vi "whereami.vi"() -> ()   [LabVIEW 2015]
uses:
  G_NAV.vi
  G_VEH.vi
  G_PATH.vi
panel:
  out "Array 2":i32[](array[numeric])
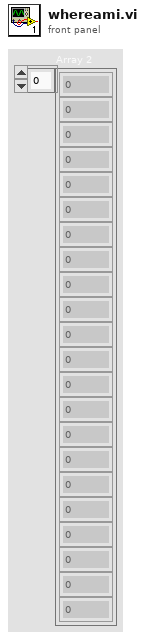
[diagram p1: front panel]
types:
  T1 = cluster{"c_idx":i32, "xc":dbl, "yc":dbl, "hc":dbl, "xc_path":dbl}
  T2 = cluster{"GPSTime":dbl, "attitude[2]":dbl, "lcc[0]":dbl, "lcc[1]":dbl, "heading_GPS":dbl}
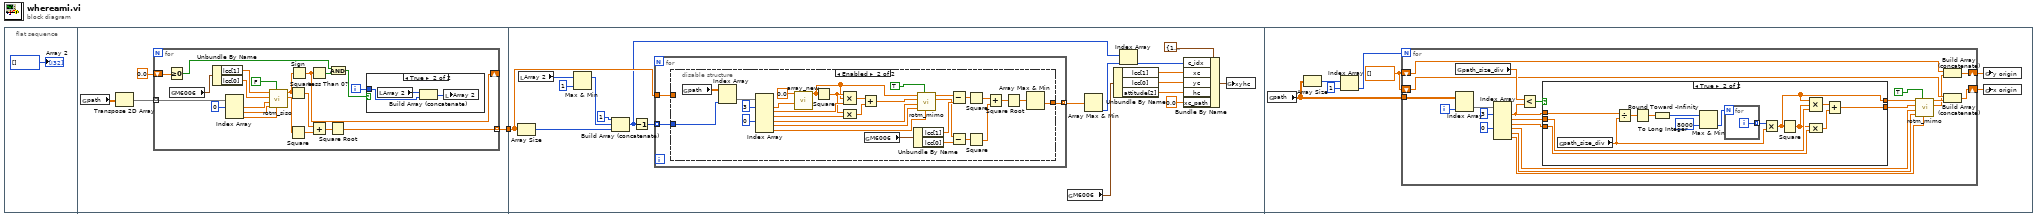
[diagram p0: block diagram]
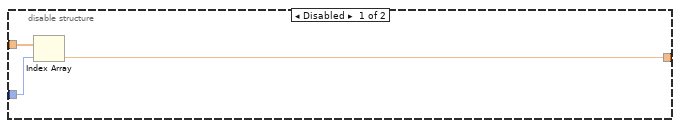
[diagram p3: hidden frame]
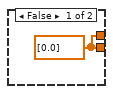
[diagram p4: hidden frame]
diagram:
  n1 = flat-sequence {
    tunnel: [w4] -> w1
    tunnel: w1 -> [w46]
    frame #0 {
      "Array 2" <- i32[] []
    }
    frame #1 {
      n2 = global read "G_PATH.vi" "path"() -> (w3:dbl[][])
      n3 = Transpose 2D Array(2D array=w3) -> (transposed array=w6:dbl[][])
      n4 = for {
        tunnel: w6 -> [w27] mode=indexing
        shift-right: [w13] -> _
        shift-left: 0.0 -> [w18]
        tunnel: [w7] -> w4 mode=indexing
        i -> [w14]
        n5 = Greater Or Equal To 0?(x=w18) -> (x >= 0?=w16:bool)
        n6 = global read "G_NAV.vi" "M6006"() -> (w25:T2)
        n7 = Unbundle By Name(w25) -> ("lcc[1]"=w24:dbl, "lcc[0]"=w23:dbl)
        n8 = Index Array(array=w27, index #1=0 ("index")) -> (element #1=w22:dbl, element #2=w21:dbl, element #3=w20:dbl)  [unwired: 2 in]
        n9 = call "rotm_siso.vi"("angle[rad]"=w20, "reverse"=FALSE, "y0"=w21, "x0"=w22, "y"=w23, "x"=w24) -> ("y'"=w11:dbl, "x'"=w12:dbl)  [unwired: 4 in]
        n10 = Square(x=w12) -> (x^2=w9:dbl)
        n11 = Square(x=w11) -> (x^2=w10:dbl)
        n12 = Sign(1:w12) -> (0:w13:dbl)
        n13 = Less Than 0?(x=w13) -> (x < 0?=w17:bool)
        n14 = Add(x=w9, y=w10) -> (x+y=w8:dbl)
        n15 = Square Root(x=w8) -> (sqrt(x)=w7:dbl)
        n16 = And(x=w16, y=w17) -> (x .and. y?=w15:bool)
        n17 = case shown="True" w15 {
          tunnel: w14 -> [_ w28]
          frame False {
          }
          frame True {
            n18 = local read "Array 2"() -> (w30:i32[])
            n19 = Build Array (concatenate)(w30, w28) -> (w29:i32[])
            n20 = local write "Array 2"(w29) -> ()
          }
        }
      }
    }
    frame #2 {
      n21 = Array Size(array=w46) -> (size(s)=w47:i32)
      n22 = local read "Array 2"() -> (w32:i32[])
      n23 = Max & Min(x=w32, y=1) -> (max(x,y)=w31:i32[])  [unwired: 1 out]
      n24 = Build Array (concatenate)(1 ("y"), w31, w47) -> (w43:i32[])
      n25 = Decrement(x=w43) -> (x-1=w45:i32[])
      n26 = for {
        tunnel: w46 -> [w51]
        tunnel: w45 -> [w50] mode=indexing
        tunnel: [w49] -> w44 mode=indexing
        n27 = disable-structure shown="Enabled" {
          disable-tunnel: w51 -> [w54 _]
          disable-tunnel: w50 -> [w53 w56]
          disable-tunnel: [w52 w59] -> w49
          frame Disabled {
            n28 = Index Array(array=w54, index=w53) -> (element=w52:dbl)
          }
          frame Enabled {
            n29 = global read "G_PATH.vi" "path"() -> (w55:dbl[][])
            n30 = Index Array(array=w55, index (col)=w56) -> (element=w84:dbl[])  [unwired: 1 in]
            n31 = Index Array(array=w84, index #1=3 ("index"), index #4=0 ("index")) -> (element #1=w81:dbl, element #2=w80:dbl, element #3=w78:dbl, element #4=w72:dbl, element #5=w71:dbl, element #6=w60:dbl)  [unwired: 4 in]
            n32 = call "array_new.vi"("end"=w81, "start"=0.0) -> ("Array"=w61:dbl[])  [unwired: 8 in, 1 out]
            n33 = Square(x=w61) -> (x^2=w79:dbl[])
            n34 = Compound Arithmetic op=MULTIPLY(w79, w61, w80) -> (w77:dbl[])
            n35 = Compound Arithmetic op=MULTIPLY(w79, w78) -> (w76:dbl[])
            n36 = Add(x=w77, y=w76) -> (x+y=w74:dbl[])
            n37 = global read "G_NAV.vi" "M6006"() -> (w70:T2)
            n38 = Unbundle By Name(w70) -> ("lcc[1]"=w69:dbl, "lcc[0]"=w68:dbl)
            n39 = call "rotm_mimo.vi"("angle[rad]"=w60, "reverse"=TRUE, "y0"=w71, "x0"=w72, "y"=w74, "x"=w61) -> ("Y"=w62:dbl[], "X"=w63:dbl[])  [unwired: 2 in, 2 out]
            n40 = Subtract(x=w63, y=w69) -> (x-y=w67:dbl[])
            n41 = Subtract(x=w62, y=w68) -> (x-y=w66:dbl[])
            n42 = Square(x=w67) -> (x^2=w65:dbl[])
            n43 = Square(x=w66) -> (x^2=w64:dbl[])
            n44 = Add(x=w65, y=w64) -> (x+y=w58:dbl[])
            n45 = Square Root(x=w58) -> (sqrt(x)=w57:dbl[])
            n46 = Array Max & Min(array=w57) -> (min value=w59:dbl)  [unwired: 3 out]
          }
        }
      }
      n47 = global read "G_NAV.vi" "M6006"() -> (w38:T2)
      n48 = Array Max & Min(array=w44) -> (min index (indices)=w42:i32)  [unwired: 3 out]
      n49 = Unbundle By Name(w38) -> ("lcc[1]"=w37:dbl, "lcc[0]"=w36:dbl, "attitude[2]"=w35:dbl)
      n50 = Index Array(array=w43, index=w42) -> (element=w39:i32)
      n51 = Bundle By Name(cluster=T1 {"c_idx"=1, "xc"=7.6063100382766855, "yc"=-606.4633590892067, "hc"=0.5767419779046403, "xc_path"=-34.68881211625345} ("xyhc"), "c_idx"=w39, "xc"=w37, "yc"=w36, "hc"=w35, "xc_path"=0.0) -> (w41:T1)
      n52 = global write "G_VEH.vi" "xyhc"(w41) -> ()
    }
    frame #3 {
      w89 = dbl[] []
      n53 = global read "G_PATH.vi" "path"() -> (w85:dbl[][])
      n54 = Array Size(array=w85) -> (size(s)=w88:i32[])
      n55 = Index Array(array=w88, index=1) -> (element=w86:i32)
      n56 = for {
        N: w86 -> [_]
        shift-right: [w97] -> w90
        shift-left: w89 -> [w99]
        shift-right: [w94] -> w91
        shift-left: w89 -> [w96]
        tunnel: w85 -> [w92]
        i -> [w93]
        n57 = global read "G_VEH.vi" "path_size_div"() -> (w108:dbl)
        n58 = Index Array(array=w92, index (col)=w93) -> (element=w113:dbl[])  [unwired: 1 in]
        n59 = Index Array(array=w113, index #1=3 ("index"), index #4=0 ("index")) -> (element #1=w107:dbl, element #2=w110:dbl, element #3=w109:dbl, element #4=w102:dbl, element #5=w101:dbl, element #6=w100:dbl)  [unwired: 4 in]
        n60 = Less?(x=w108, y=w107) -> (x < y?=w111:bool)
        n61 = case shown="True" w111 {
          tunnel: w107 -> [_ w129]
          tunnel: w110 -> [_ w124]
          tunnel: w109 -> [_ w123]
          tunnel: [w114 w119] -> w106
          tunnel: [w114 w118] -> w105
          frame False {
            w114 = dbl[] [0.0]
          }
          frame True {
            n62 = global read "G_VEH.vi" "path_size_div"() -> (w125:dbl)
            n63 = Divide(x=w129, y=w125) -> (x/y=w128:dbl)
            n64 = Round Toward -Infinity(1:w128) -> (0:w127:dbl)
            n65 = To Long Integer(number=w127) -> (32bit integer=w116:i32)
            n66 = Max & Min(x=w116, y=8000) -> (min(x,y)=w115:i32)  [unwired: 1 out]
            n67 = for {
              N: w115 -> [_]
              tunnel: [w130] -> w126 mode=indexing
              i -> [w130]
            }
            n68 = Multiply(x=w126, y=w125) -> (x*y=w119:dbl[])
            n69 = Square(x=w119) -> (x^2=w120:dbl[])
            n70 = Compound Arithmetic op=MULTIPLY(w119, w120, w124) -> (w122:dbl[])
            n71 = Compound Arithmetic op=MULTIPLY(w120, w123) -> (w121:dbl[])
            n72 = Add(x=w122, y=w121) -> (x+y=w118:dbl[])
          }
        }
        n73 = call "rotm_mimo.vi"("angle[rad]"=w100, "reverse"=TRUE, "y0"=w101, "x0"=w102, "y"=w105, "x"=w106) -> ("Y"=w95:dbl[], "X"=w98:dbl[])  [unwired: 2 in, 2 out]
        n74 = Build Array (concatenate)(w96, w95) -> (w94:dbl[])
        n75 = Build Array (concatenate)(w99, w98) -> (w97:dbl[])
      }
      n76 = global write "G_PATH.vi" "y origin"(w91) -> ()
      n77 = global write "G_PATH.vi" "x origin"(w90) -> ()
    }
  }
